vi "editDialog.vi"(0 "reference":refnum<class "PackageNode.lvclass">, 1 "insidePackageNode":bool, 5 "error in (no error)":errorcluster) -> (14 "reference out":refnum<class "PackageNode.lvclass">, 15 "changeConnection":T1, 16 "cancel":bool, 19 "error out":errorcluster)   [LabVIEW 2016, in "PackageNode.lvclass"]
doc: "Edit Dialog"
uses:
  <resource>/Framework/Providers/Open_GDS/UML/PackageNode_class/PackageNode.lvclass
  C:/Program Files (x86)/National Instruments/LabVIEW 2016/resource/Framework/Providers/Open_GDS/UML/AbstractNode_class/AbstractNode.lvclass
  <resource>/Framework/Providers/Open_GDS/UML/AbstractNode_class/private/NodeConnectionStatsType.ctl
  <resource>/Framework/Providers/Open_GDS/UML/ContextHelp/ContextHelp_HelpTexts.ctl
  <resource>/Framework/Providers/Open_GDS/UML/MultiLineString_class/JustificationType.ctl
  <resource>/Framework/Providers/Open_GDS/UML/MultiLineString_class/MultiLineString.lvclass
  <resource>/Framework/Providers/Open_GDS/UML/AbstractNode_class/AbstractNode.lvclass
panel:
  in  "Justification":u16(ring) items=["Center", "Top left corner"]
  in  "Package color":u32(colorbox)
  in  "connection":bool caption="Connect to Package"
  in  "Help":bool
  in  "Package Name":string
  in  "Text":string
  in  "Cancel Button":bool
  in  "OK Button":bool
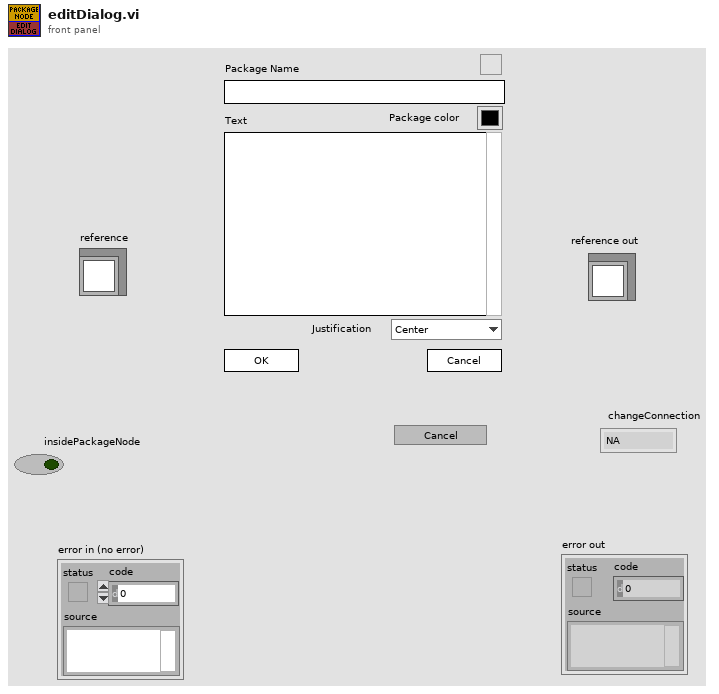
[diagram p1: front panel]
types:
  T1 = typedef "AbstractNode.lvclass/NodeConnectionStatsType.ctl" = enum16{"NA", "Connect", "DisConnect"}
  T2 = typedef "ContextHelp_HelpTexts.ctl" = enum16{"None(Hide)", "Default", "Help", "Welcome", "GettingStarted", "ClassDiagram_Help", "SequenceDiagram_Help", "UseCaseDiagram_Help", "BSelect", "BClass", "BInterface", "BPackage", "BNote", "BDependency", "BInheritance", "BInterfaceImplementation", "BAssociation", "BAggregation", "BCompAggregation", "BNoteConnector", "BObject", "BActionBar", "BCall", "BSystem", "BActor", "BUseCase", "BGeneralization", "BIncludes", "BExtends", "BUseCaseDiagramAssociation", "ClassRelationshipEdge editDialog_Bent Style", "ClassRelationshipEdge editDialog_RelationType", "ClassRelationshipEdge editDialog_Reverse association", "ClassRelationshipEdge editDialog_Start label", "ClassRelationshipEdge editDialog_Middle label", "ClassRelationshipEdge editDialog_End label", "UMLEditor reversedEngineering_Pathes", "ReversedEngineering StateReverseDialog_Help", "ReversedEngineering StateQueuedSettings_Help", "UMLEditor reversedEngineering_AddTopVIs", "UMLEditor reversedEngineering_AddClasses", "UMLEditor reversedEngineering_AddDirs", "UMLEditor reversedEngineering_Recursively", "UMLEditor reversedEngineering_Remove", "UMLEditor reversedEngineering_ClearList", "UMLEditor reversedEngineering_HideSubAss", "UMLEditor reversedEngineering_CreateTypes", "UMLEditor reversedEngineering_OnlyInheritance", "UMLEditor reversedEngineering_CreateApplication", "UMLEditor reversedEngineering_OK", "UMLEditor reversedEngineering_Cancel", "UMLEditor reversedEngineering_Help", "UMLEditor createWizardScriptFile_ScriptfilePath", "UMLEditor createWizardScriptFile_ClassPath", "UMLEditor createWizardScriptFile_Use", "UMLEditor createWizardScriptFile_PrivateDirName", "UMLEditor createWizardScriptFile_DirAppend", "UMLEditor createWizardScriptFile_Separator Character", "UMLEditor createWizardScriptFile_OK", "UMLEditor createWizardScriptFile_Cancel", "UMLEditor createWizardScriptFile_Help", "ClassNode editDialog_Class Name", "InterfaceNode editDialog_Class Name", "ClassNode editDialog_Attribute", "ClassNode editDialog_Methods", "InterfaceNode editDialog_Methods", "ClassNode editDialog_connection", "InterfaceNode editDialog_connection", "ClassNode editDialog_StereoType", "ClassNode editDialog_ShowAttrib", "ClassNode editDialog_ShowMethods", "ClassNode editDialog_ClassPath", "ClassNode editDialog_AddAttribute", "ClassNode editDialog_AddMethod", "InterfaceNode editDialog_AddMethod", "ClassNode AttributeGuide_AttributeName", "ClassNode AttributeGuide_Array?", "ClassNode AttributeGuide_Data Type", "ClassNode AttributeGuide_RefName", "ClassNode AttributeGuide_Preview", "ClassNode AttributeGuide_OK", "ClassNode AttributeGuide_Cancel", "ClassNode MethodGuide_Visibility", "ClassNode MethodGuide_Method Name", "ClassNode MethodGuide_Preview", "ClassNode MethodGuide_OK", "ClassNode MethodGuide_Cancel", "CallNode EditCallProperties_AllButtons", "ObjectNode EditObjectlProperties_AllButtons", "ActorNode EditActorProperties_AllButtons", "UseCaseRelationshipNode EditUseCaselProperties_AllButtons", "UseCaseNode EditUseCaselProperties_AllButtons", "SystemNode EditSystemProperties_AllButtons", "ReversedEngineering UpdateAttributes_AllButtons", "StateNode editDialog_AllButtons", "StateTransition editDialog_AllButtons", "ArrangeNodes Main_Picture", "ArrangeNodes Main_Zoom", "ArrangeNodes Main_Auto Zoom", "ArrangeNodes Main_shorten", "ArrangeNodes Main_Min Length", "ArrangeNodes Main_Max Length", "ArrangeNodes Main_increase", "ArrangeNodes Main_decrease", "ArrangeNodes Main_Shake", "ArrangeNodes Main", "BState", "BInitialState", "BFinalState", "BStateTransition", "StateDiagram_Help", "StateDiagram_PropertiesAllButtons", "ReversedEngineering StateReverseDialog_ClearStates", "ReversedEngineering StateReverseDialog_UseQueuedStateMachines", "ReversedEngineering StateReverseDialog_QueuedSettings", "ReversedEngineering StateReverseDialog_SearchForVIs", "ReversedEngineering StateReverseDialog_SearchCriteria", "OptionsDialog_ClassBasePath", "OptionsDialog_VIPath", "OptionsDialog_ApplicationPath", "OptionsDialog_WizDir", "OptionsDialog_IniFilePath", "OptionsDialog_DefineColors", "OptionsDialog_Help", "OptionsDialog_CreateTypes", "ClassRelationshipEdge editDialog_SplitWire"}
  T3 = typedef "MultiLineString.lvclass/JustificationType.ctl" = enum16{"LEFT", "CENTER", "RIGHT"}
  T4 = typedef "ContextHelp_ShowType.ctl" = cluster{"Header":string, "Picture":picture, "Text":string}
  T5 = typedef "PackageNode.lvclass/ObjectAttributes.ctl" = cluster{"name":string, "contents":refnum<class "MultiLineString.lvclass">, "DEFAULT_TOP_WIDTH":i32, "DEFAULT_TOP_HEIGHT":i32, "DEFAULT_WIDTH":i32, "DEFAULT_HEIGHT":i32, "NAME_GAP":i32, "XGAP":i32, "YGAP":i32, "Collapsed":bool, "Note color":u32, "Justification":u16}
  T6 = typedef "AbstractNode.lvclass/ObjectAttributes.ctl" = cluster{"parent":refnum<class "AbstractNode.lvclass">, "children":refnum<class "AbstractNode.lvclass">[], "Hidden":bool}
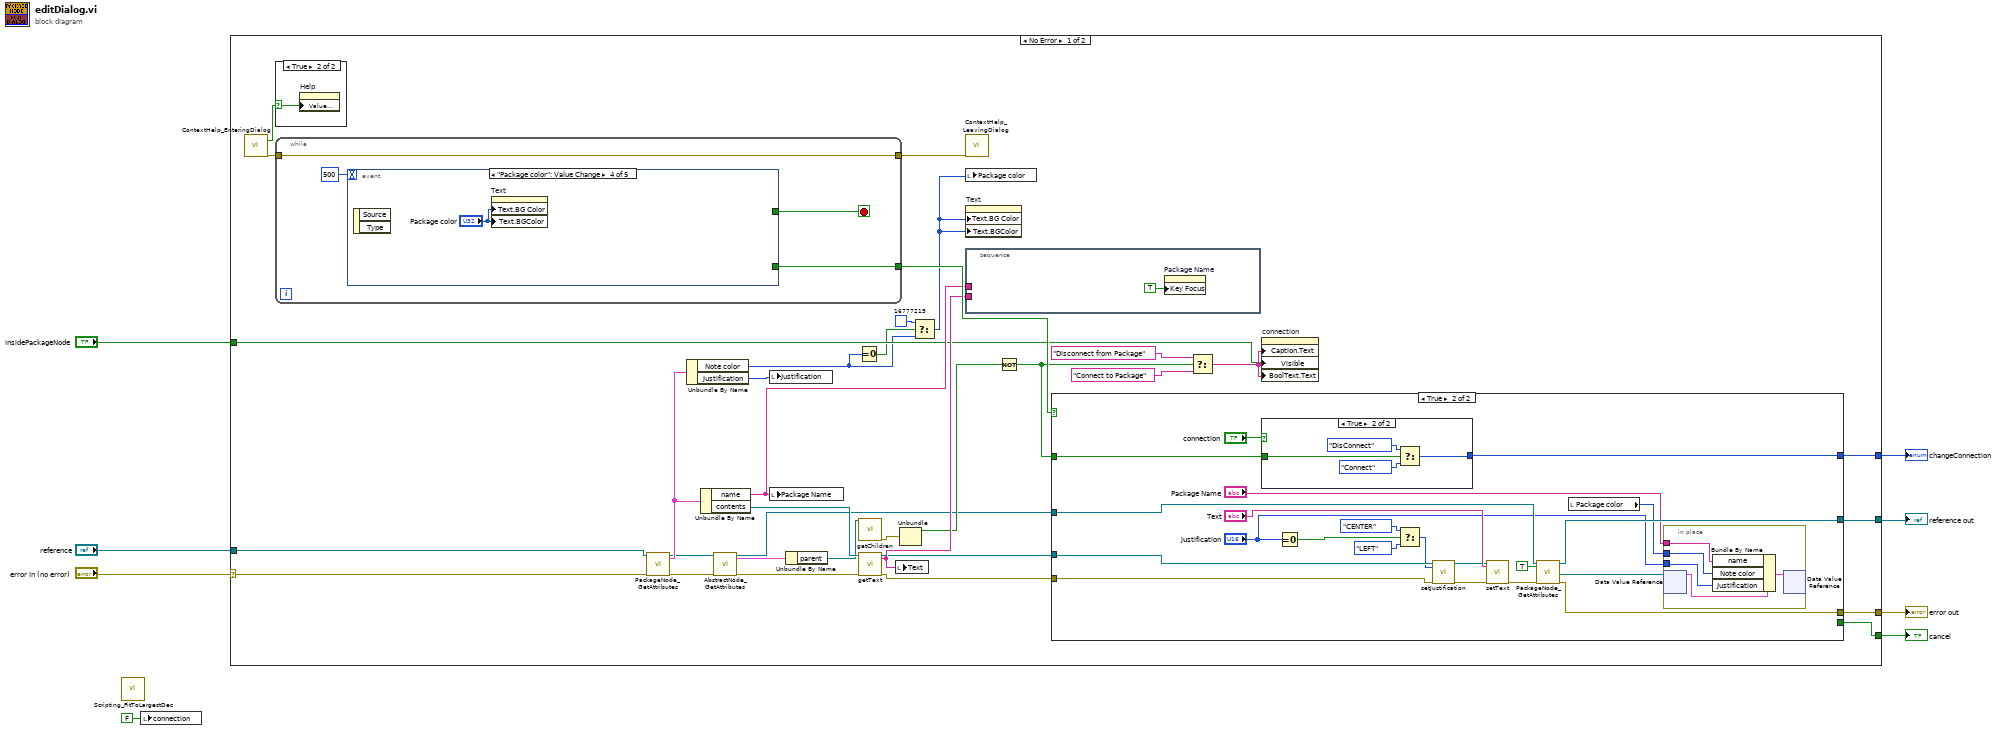
[diagram p0: block diagram]
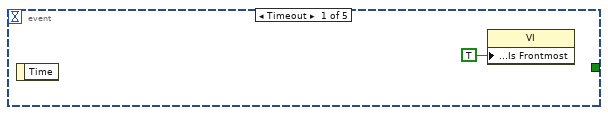
[diagram p3: hidden frame]
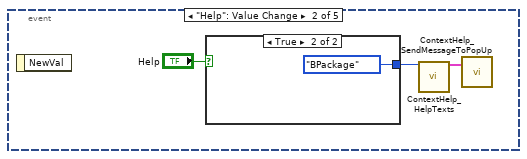
[diagram p4: hidden frame]
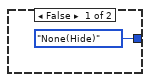
[diagram p5: hidden frame]
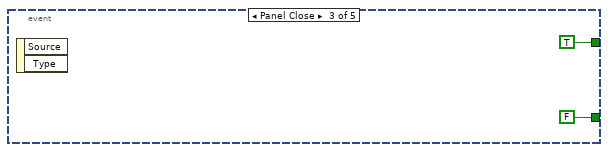
[diagram p6: hidden frame]
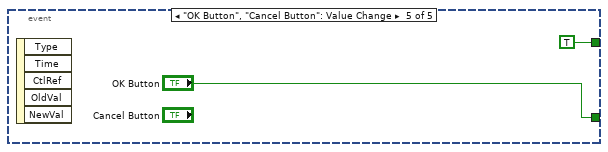
[diagram p7: hidden frame]
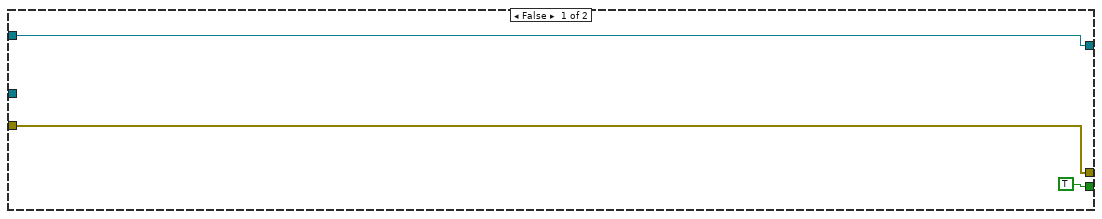
[diagram p8: hidden frame]
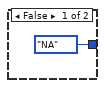
[diagram p9: hidden frame]
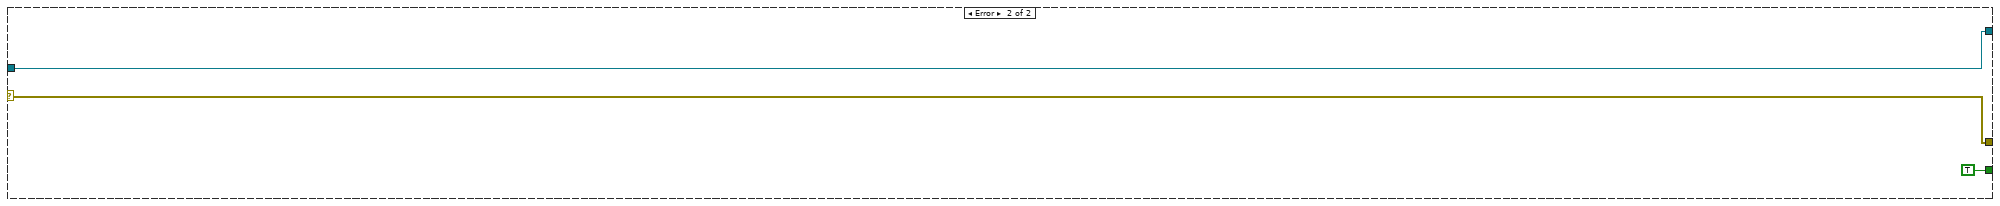
[diagram p10: hidden frame]
diagram:
  n1 = call <resource>:"Scripting_FitToLargestDec.vi"() -> ()  [unwired: 6 in, 2 out]
  n2 = local write "connection"(FALSE ("connection")) -> ()
  n3 = case shown="No Error" "error in (no error)" {
    selector: "error in (no error)" -> [w39 w95]
    tunnel: "reference" -> [w40 w96]
    tunnel: [w42 w95] -> w6
    tunnel: [w41 w96] -> w5
    tunnel: [w32 TRUE ("Key Focus")] -> w4
    tunnel: [w28 _] -> w3
    tunnel: "insidePackageNode" -> [w21 _]
    frame No Error {
      n4 = call <resource>:"ContextHelp_EnteringDialog.vi"() -> ("HelpStatus"=w29:bool, "error out"=w31:errorcluster)  [unwired: 3 in, 15 out]
      n5 = case shown="True" w29 {
        selector: w29 -> [_ w43]
        frame False {
        }
        frame True {
          n6 = property on="Help" class="Bool (strict)"("Value (Signaling)"=w43) -> ()  [unwired: 2 in, 2 out]
        }
      }
      n7 = while {
        tunnel: [w47] -> w38
        tunnel: w31 -> [w46]
        tunnel: [w46] -> w30
        stop <- w44 stop-if-true
        n8 = event shown="[3] \"Package color\": Value Change" {
          selector: _ -> [_ _ _ _ _]
          dyn-events: _ -> [_ _ _ _ _]
          timeout: 500 -> [_ _ _ _ _]
          tunnel: [_ _ FALSE ("OK Button") _ "OK Button"] -> w47
          tunnel: [_ _ TRUE ("Front Panel Window:Is Frontmost") _ TRUE] -> w44
          event Timeout {
            n9 = event-data() -> ()  [unwired: 2 out]
            n10 = property class="VI"("Front Panel Window:Is Frontmost"=TRUE) -> ()  [unwired: 2 in, 2 out]
          }
          event "Help": Value Change {
            n11 = event-data() -> ()  [unwired: 2 out]
            n12 = case shown="True" "Help" {
              tunnel: [ContextHelp_HelpTexts."None(Hide)" ("HelpText") ContextHelp_HelpTexts."BPackage" ("HelpText")] -> w50
              frame False {
              }
              frame True {
              }
            }
            n13 = call <resource>:"ContextHelp_HelpTexts.vi"("HelpText (enum or string)"=w50) -> ("HelpOut"=w51:T4)  [unwired: 18 out]
            n14 = call <resource>:"ContextHelp_SendMessageToPopUp.vi"("PopUpMessage"=w51) -> ()  [unwired: 2 in, 17 out]
          }
          event Panel Close {
            n15 = event-data() -> ()  [unwired: 3 out]
          }
          event "Package color": Value Change {
            n16 = event-data() -> ()  [unwired: 3 out]
            n17 = property on="Text" class="Str"("Text.BG Color"="Package color", "Text.BGColor"="Package color") -> ()  [unwired: 2 in, 2 out]
          }
          event "OK Button", "Cancel Button": Value Change {
            n18 = event-data() -> ()  [unwired: 6 out]
          }
        }
      }
      n19 = call <resource>:"PackageNode_GetAttributes.vi"("reference in"=w40, "error in (no error)"=w39) -> ("reference out"=w13:refnum<class "PackageNode.lvclass">, "Data"=w14:T5, "error out"=w12:errorcluster)  [unwired: 1 in, 14 out]
      n20 = Unbundle By Name(w14) -> ("Note color"=w17:u32, "Justification"=w19:u16)
      n21 = Unbundle By Name(w14) -> ("name"=w33:string, "contents"=w37:refnum<class "MultiLineString.lvclass">)
      n22 = call <resource>:"AbstractNode_GetAttributes.vi"("reference in"=w13, "error in (no error)"=w12) -> ("reference out"=w10:refnum<class "PackageNode.lvclass">, "Data"=w9:T6, "error out"=w11:errorcluster)  [unwired: 14 in, 1 out]
      n23 = local write "Justification"(w19) -> ()
      n24 = local write "Package Name"(w33) -> ()
      n25 = Unbundle By Name(w9) -> ("parent"=w26:refnum<class "AbstractNode.lvclass">)
      n26 = Equal To 0?(x=w17) -> (x = 0?=w18:bool)
      n27 = call-dynamic "getChildren.vi"("reference"=w26) -> ("error out"=w24:errorcluster)  [unwired: 15 in, 3 out]
      n28 = call-dynamic "getText.vi"("reference"=w37, "error in (no error)"=w11) -> ("reference out"=w35:refnum<class "MultiLineString.lvclass">, "text"=w36:string, "error out"=w34:errorcluster)  [unwired: 15 in]
      n29 = local write "Text"(w36) -> ()
      n30 = Unbundle(w24) -> ("status"=w25:bool)  [unwired: 2 out]
      n31 = Select(t=u32 16777215, s=w18, f=w17) -> (s? t:f=w16:u32)
      n32 = call <resource>:"ContextHelp_LeavingDialog.vi"("error in (no error)"=w30) -> ()  [unwired: 2 in, 17 out]
      n33 = local write "Package color"(w16) -> ()
      n34 = property on="Text" class="Str"("Text.BG Color"=w16, "Text.BGColor"=w16) -> ()  [unwired: 2 in, 2 out]
      n35 = stacked-sequence {
        tunnel: w33 -> [_]
        tunnel: w36 -> [_]
        frame #0 {
          n36 = property on="Package Name" class="Str"("Key Focus"=TRUE) -> ()  [unwired: 2 in, 2 out]
        }
      }
      n37 = Not(x=w25) -> (.not. x?=w20:bool)
      n38 = case shown="True" w38 {
        tunnel: [w60 w82] -> w42
        tunnel: [w61 w81] -> w41
        tunnel: w10 -> [w61 w80]
        tunnel: w35 -> [_ w72]
        tunnel: w34 -> [w60 w74]
        tunnel: [TRUE ("Key Focus") _] -> w32
        tunnel: [_ w76] -> w28
        tunnel: w20 -> [_ w75]
        frame False {
        }
        frame True {
          n39 = case shown="True" "connection" {
            tunnel: [enum16{"NA", "Connect", "DisConnect"}."NA" ("changeConnection") w91] -> w76
            tunnel: w75 -> [_ w92]
            frame False {
            }
            frame True {
              n40 = Select(t=enum16{"NA", "Connect", "DisConnect"}."DisConnect" ("changeConnection"), s=w92, f=enum16{"NA", "Connect", "DisConnect"}."Connect" ("changeConnection")) -> (s? t:f=w91:enum16{"NA", "Connect", "DisConnect"})
            }
          }
          n41 = Equal To 0?(x="Justification") -> (x = 0?=w70:bool)
          n42 = Select(t=JustificationType."CENTER" ("justification"), s=w70, f=JustificationType."LEFT" ("justification")) -> (s? t:f=w67:T3)
          n43 = call <resource>:"setJustification.vi"("reference"=w72, "justification"=w67, "error in (no error)"=w74) -> ("reference out"=w71:refnum<class "MultiLineString.lvclass">, "error out"=w73:errorcluster)  [unwired: 15 in]
          n44 = call-dynamic "setText.vi"("reference"=w71, "text"="Text", "error in (no error)"=w73) -> ("error out"=w78:errorcluster)  [unwired: 15 in, 1 out]
          n45 = call <resource>:"PackageNode_GetAttributes.vi"("reference in"=w80, "OnlyGetDvrReference(False)"=TRUE, "error in (no error)"=w78) -> ("reference out"=w81:refnum<class "PackageNode.lvclass">, "DataRef"=w65:refnum<data-value>, "error out"=w82:errorcluster)  [unwired: 13 in, 1 out]
          n46 = local read "Package color"() -> (w63:u32)
          n47 = in-place {
            in-place-border: "Package Name" -> [w86]
            in-place-border: w63 -> [w85]
            in-place-border: "Justification" -> [w84]
            n48 = in-place-dvr #1(w65) -> (w87:T5)  [unwired: 1 out]
            n49 = Bundle By Name(cluster=w87, "name"=w86, "Note color"=w85, "Justification"=w84) -> (w83:T5)
            n50 = in-place-dvr #1(w83) -> ()  [unwired: 2 out]
          }
        }
      }
      n51 = Select(t="Disconnect from Package", s=w20, f="Connect to Package") -> (s? t:f=w27:string)
      n52 = property on="connection" class="Bool (strict)"("Caption.Text"=w27, "Visible"=w21, "BoolText.Text"=w27) -> ()  [unwired: 2 in, 2 out]
    }
    frame Error {
    }
  }
  "reference out" <- w5
  "error out" <- w6
  "changeConnection" <- w3
  "cancel" <- w4
